vi "Scale.vi"(9 "Numeric 3":u32, 10 "Redness":dbl, 11 "Numeric in":u32) -> (3 "Numeric out":dbl)   [LabVIEW 2014]
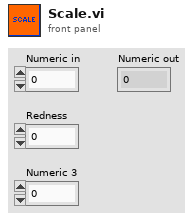
[diagram p1: front panel]
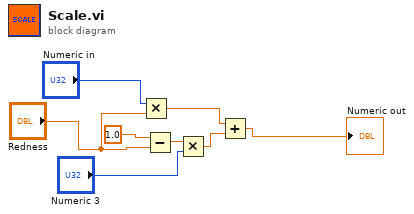
[diagram p0: block diagram]
diagram:
  n1 = Multiply(x="Numeric in", y="Redness") -> (x*y=w6:dbl)
  n2 = Subtract(x=1.0, y="Redness") -> (x-y=w4:dbl)
  n3 = Multiply(x=w4, y="Numeric 3") -> (x*y=w5:dbl)
  n4 = Add(x=w6, y=w5) -> (x+y=→"Numeric out":dbl)
